vi "GV pixel clock.vi"() -> ()   [LabVIEW 2017]
panel:
  out "Pixel clock":bool
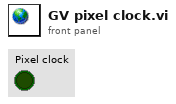
[diagram p1: front panel]
diagram:
